vi "GateIncrement.vi"(9 "Voltage Safety Limit":dbl=7.0, 10 "Increment":dbl=0.09999999999999999, 11 "Gate Voltage":dbl) -> ()   [LabVIEW 2021]
panel:
  in  "Stop":bool
  # "Gate Increment"
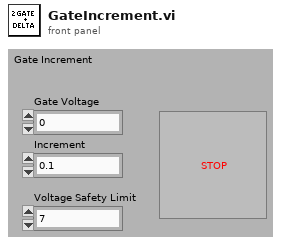
[diagram p1: front panel]
types:
  T1 = enum16{"Set Voltage", "Read Voltage", "Read Current", "Output On", "Output Off", "Set Increment", "Set Increment Time", "Stop Voltage Set", "Set Maximum Voltage", "Get Maximum Voltage"}
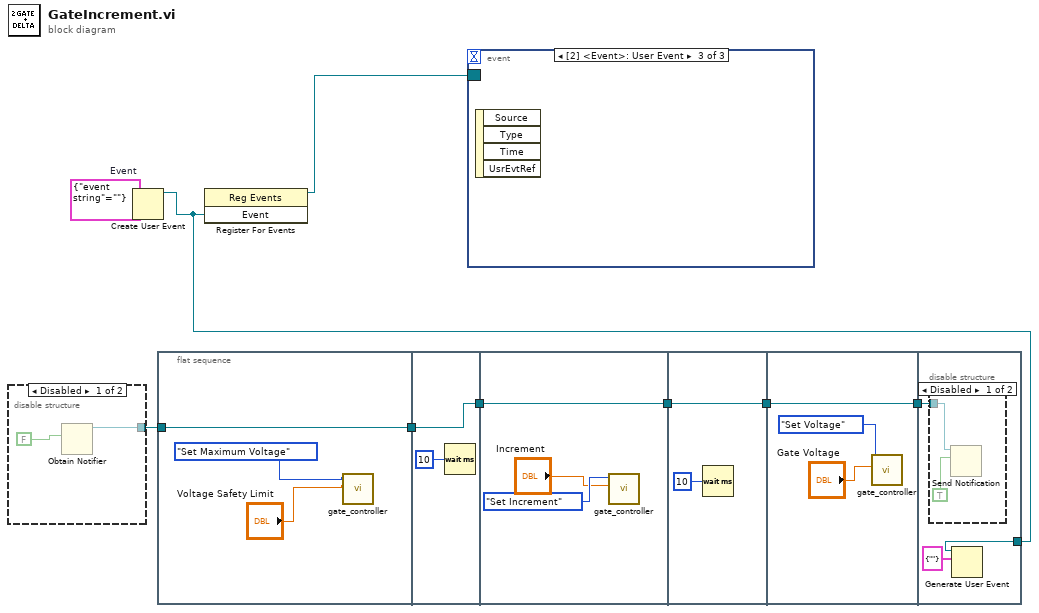
[diagram p0: block diagram]
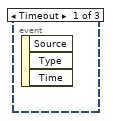
[diagram p3: hidden frame]
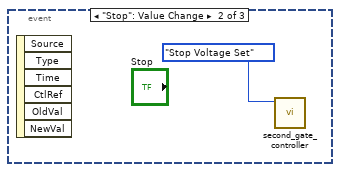
[diagram p4: hidden frame]
diagram:
  w1 = cluster{"event string":string} {"event string"=""}  # Event
  n1 = disable-structure shown="Disabled" {
    disable-tunnel: [w10 _] -> w4
    frame Disabled {
      n2 = Obtain Notifier(notification data type=FALSE) -> (notifier out=w10:refnum<notifier>)  [unwired: 3 in, 2 out]
    }
    frame Enabled {
    }
  }
  n3 = Create User Event(user event datatype=w1) -> (user event=w2:refnum<user-event>)  [unwired: 1 in, 1 out]
  n4 = flat-sequence {
    tunnel: w4 -> [w14]
    tunnel: [w14] -> w9
    tunnel: w9 -> [w15]
    tunnel: [w15] -> w8
    tunnel: w8 -> [w19]
    tunnel: [w19] -> w7
    tunnel: w7 -> [w20]
    tunnel: [w20] -> w6
    tunnel: w6 -> [w24]
    tunnel: [w24] -> w5
    tunnel: w5 -> [w27]
    tunnel: w2 -> [w26]
    frame #0 {
      n5 = call "gate_controller.vi"("Numerical Argument"="Voltage Safety Limit", "Command"=T1."Set Maximum Voltage") -> ()  [unwired: 9 in, 1 out]
    }
    frame #1 {
      n6 = Wait (ms)(milliseconds to wait=u32 10) -> ()  [unwired: 1 out]
    }
    frame #2 {
      n7 = call "gate_controller.vi"("Numerical Argument"="Increment", "Command"=T1."Set Increment") -> ()  [unwired: 9 in, 1 out]
    }
    frame #3 {
      n8 = Wait (ms)(milliseconds to wait=u32 10) -> ()  [unwired: 1 out]
    }
    frame #4 {
      n9 = call "gate_controller.vi"("Numerical Argument"="Gate Voltage", "Command"=T1."Set Voltage") -> ()  [unwired: 9 in, 1 out]
    }
    frame #5 {
      n10 = disable-structure shown="Disabled" {
        disable-tunnel: w27 -> [w29 _]
        frame Disabled {
          n11 = Send Notification(notification=TRUE, notifier=w29) -> ()  [unwired: 1 in, 2 out]
        }
        frame Enabled {
        }
      }
      n12 = Generate User Event(user event=w26, event data cluster=cluster{string} {""} ("event data")) -> ()  [unwired: 2 in, 2 out]
    }
  }
  n13 = register-events(w2) -> (reference out=w3:refnum<event-registration>)  [unwired: 2 in, 1 out]
  n14 = event shown="[2] <Event>: User Event" {
    selector: w3 -> [_ _ _]
    dyn-events: _ -> [_ _ _]
    timeout: _ -> [_ _ _]
    event Timeout {
      n15 = event-data() -> ()  [unwired: 1 in, 3 out]
    }
    event "Stop": Value Change {
      n16 = event-data() -> ()  [unwired: 1 in, 6 out]
      n17 = call "second_gate_controller.vi"("Command"=T1."Stop Voltage Set") -> ()  [unwired: 10 in, 1 out]
    }
    event User Event {
      n18 = event-data() -> ()  [unwired: 1 in, 4 out]
    }
  }
